vi "New_User Management (Subvi) (TR).vi"() -> ()   [LabVIEW 2009]
uses:
  <vilib>/Utility/file.llb/Read From Spreadsheet File (string).vi
  <vilib>/Utility/file.llb/Write To Spreadsheet File (string).vi
panel:
  in  "Encode/Decode":bool=TRUE
  in  "Magnitude of Shift":u8=22
  in  "Change":bool
  in  "Delete":bool
  in  "Multicolumn Listbox":i32(listbox)
  in  "Yetki":string(combo)="Öğrenci"
  in  "stop":bool
  in  "Create":bool
  in  "Şifre":string
  in  "Kullanıcı Adı":string
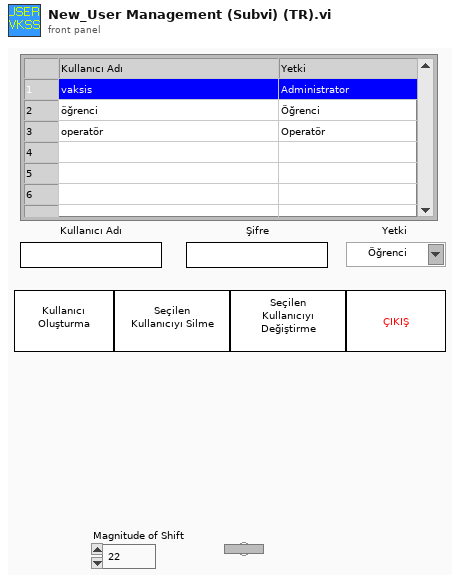
[diagram p1: front panel]
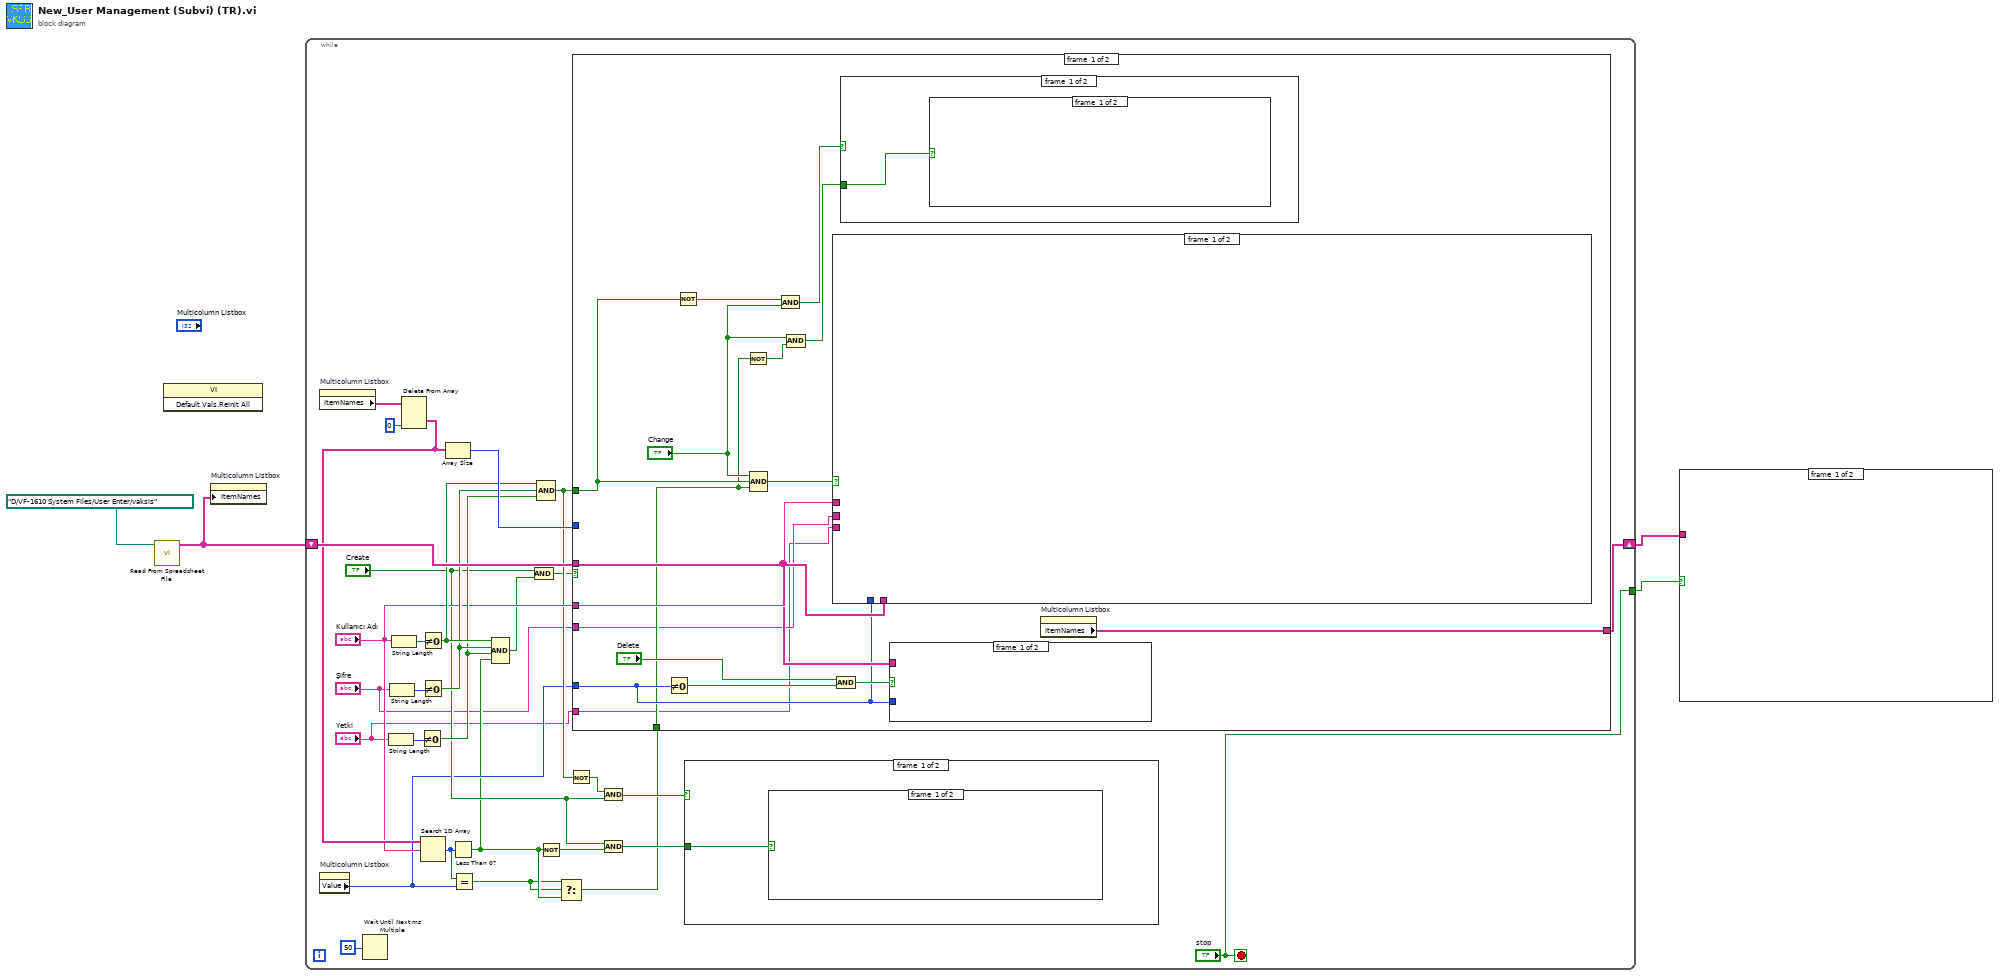
[diagram p0: block diagram]
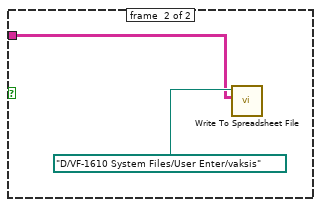
[diagram p2: hidden frame]
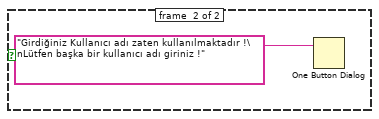
[diagram p3: hidden frame]
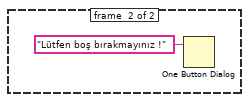
[diagram p4: hidden frame]
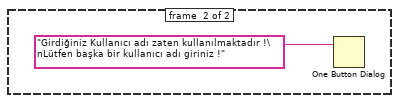
[diagram p5: hidden frame]
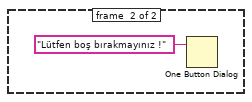
[diagram p6: hidden frame]
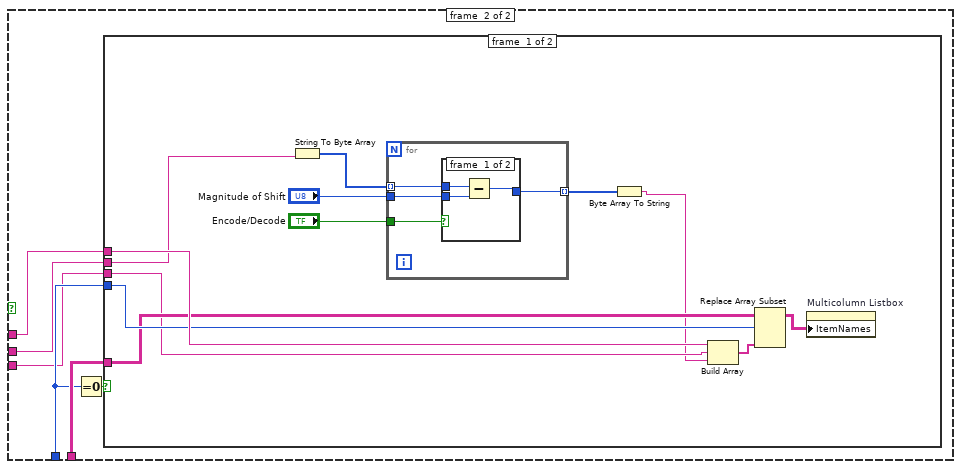
[diagram p7: hidden frame]
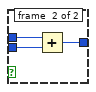
[diagram p8: hidden frame]
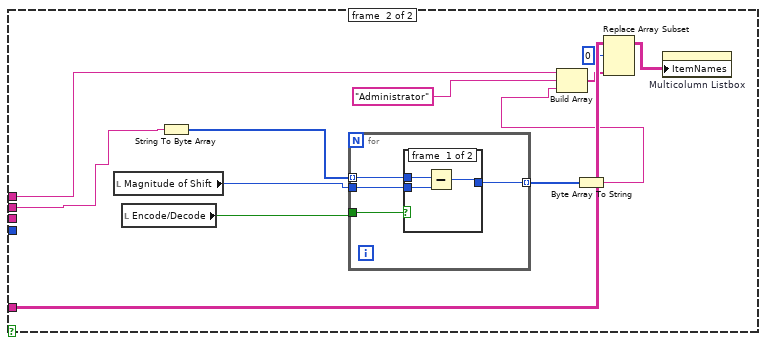
[diagram p9: hidden frame]
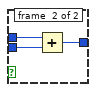
[diagram p10: hidden frame]
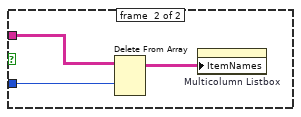
[diagram p11: hidden frame]
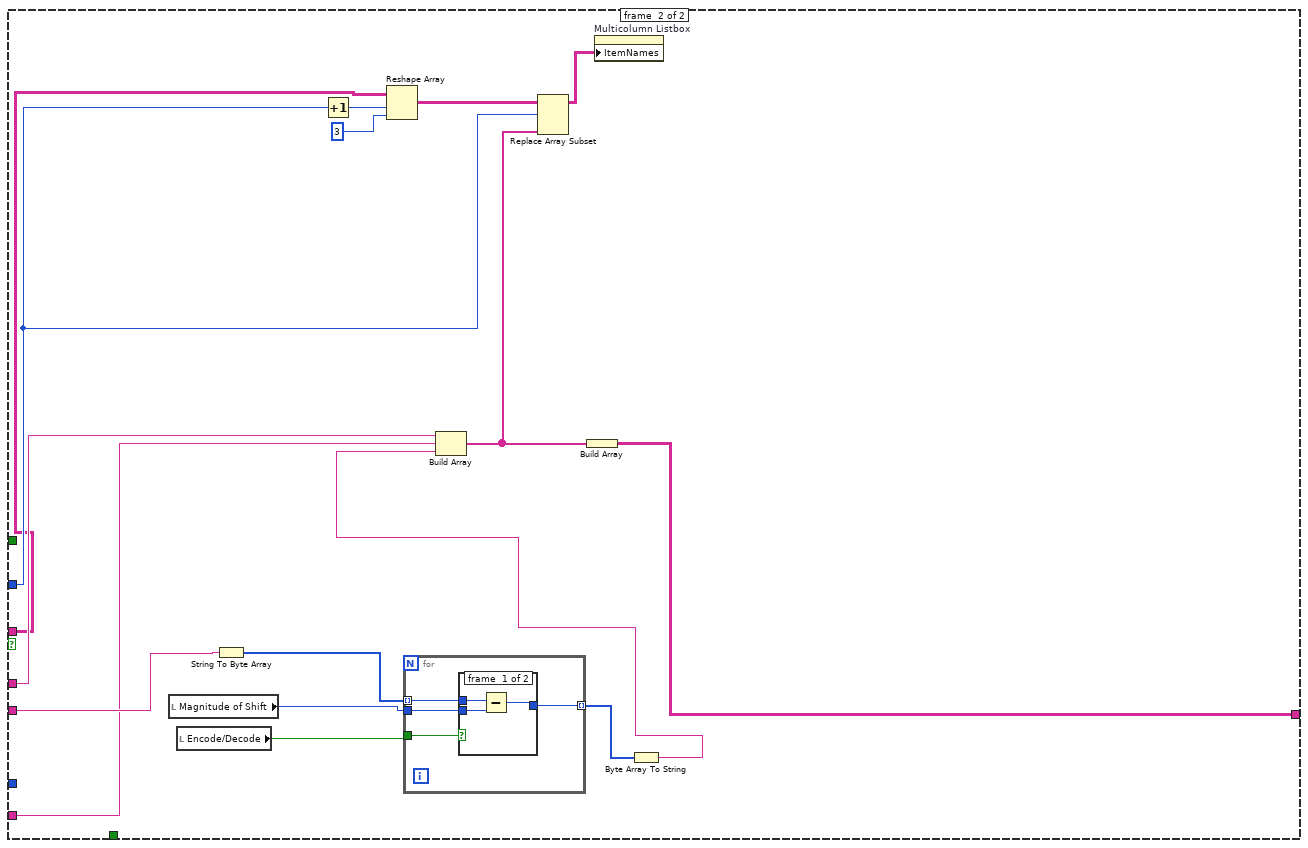
[diagram p12: hidden frame]
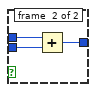
[diagram p13: hidden frame]
diagram:
  n1 = call-poly <vilib>:"Read From Spreadsheet File.vi"("file path (dialog if empty)"=path "D:/VF-1610 System Files/User Enter/vaksis" ("file (use dialog) 2")) -> ("all rows"=w1:string[][])  [unwired: 6 in, 4 out]
  n2 = invoke class="VI" method="Default Vals.Reinit All"() -> ()  [unwired: 3 in, 3 out]
  n3 = property on="Multicolumn Listbox" class="MCListbox (strict)"("ItemNames"=w1) -> ()  [unwired: 2 in, 2 out]
  n4 = while {
    shift-right: [w30] -> w3
    shift-left: w1 -> [w32]
    tunnel: ["stop"] -> w2
    stop <- "stop" stop-if-true
    n5 = property on="Multicolumn Listbox" class="MCListbox (strict)"() -> ("ItemNames"=w25:string[][])  [unwired: 2 in, 2 out]
    n6 = property on="Multicolumn Listbox" class="MCListbox (strict)"() -> ("Value"=w10:i32)  [unwired: 2 in, 2 out]
    n7 = Wait Until Next ms Multiple(millisecond multiple=u32 50) -> ()  [unwired: 1 out]
    n8 = String Length(string="Yetki") -> (length=w28:i32)
    n9 = String Length(string="Şifre") -> (length=w27:i32)
    n10 = String Length(string="Kullanıcı Adı") -> (length=w29:i32)
    n11 = Delete From Array(array=w25, index (col)=0 ("disabled index (col)")) -> (deleted portion=w20:string[])  [unwired: 2 in, 1 out]
    n12 = Not Equal To 0?(x=w28) -> (x != 0?=w21:bool)
    n13 = Not Equal To 0?(x=w29) -> (x != 0?=w23:bool)
    n14 = Not Equal To 0?(x=w27) -> (x != 0?=w22:bool)
    n15 = Search 1D Array(1D array=w20, element="Kullanıcı Adı") -> (index of element=w11:i32)  [unwired: 1 in]
    n16 = Array Size(array=w20) -> (size(s)=w24:i32)
    n17 = Less Than 0?(x=w11) -> (x < 0?=w9:bool)
    n18 = Equal?(x=w11, y=w10) -> (x = y?=w8:bool)
    n19 = Compound Arithmetic op=AND(w23, w22, w21, w9) -> (w13:bool)
    n20 = And(x="Create", y=w13) -> (x .and. y?=w14:bool)
    n21 = Compound Arithmetic op=AND(w23, w22, w21) -> (w18:bool)
    n22 = Not(x=w9) -> (.not. x?=w17:bool)
    n23 = Select(t=w8, s=w8, f=w9) -> (s? t:f=w7:bool)
    n24 = Not(x=w18) -> (.not. x?=w26:bool)
    n25 = case shown="False" w14 {
      tunnel: w24 -> [_ w122]
      tunnel: [w53 w123] -> w30
      tunnel: w32 -> [w52 w119]
      tunnel: "Kullanıcı Adı" -> [w54 w126]
      tunnel: "Yetki" -> [w38 w112]
      tunnel: "Şifre" -> [w39 w113]
      tunnel: w18 -> [w42 _]
      tunnel: w10 -> [w43 _]
      tunnel: w7 -> [w41 _]
      frame #0 {
        n26 = Not Equal To 0?(x=w43) -> (x != 0?=w49:bool)
        n27 = Not(x=w42) -> (.not. x?=w47:bool)
        n28 = Not(x=w41) -> (.not. x?=w40:bool)
        n29 = Compound Arithmetic op=AND("Change", w42, w41) -> (w51:bool)
        n30 = Compound Arithmetic op=AND(w47, "Change") -> (w46:bool)
        n31 = Compound Arithmetic op=AND("Change", w40) -> (w44:bool)
        n32 = case shown="True" w51 {
          tunnel: w52 -> [_ w62]
          tunnel: w54 -> [_ w61]
          tunnel: w39 -> [_ w60]
          tunnel: w43 -> [_ w59]
          tunnel: w38 -> [_ w58]
          frame #0 {
          }
          frame #1 {
            n33 = Equal To 0?(x=w59) -> (x = 0?=w63:bool)
            n34 = case shown="True" w63 {
              tunnel: w61 -> [w73 w93]
              tunnel: w60 -> [w66 w89]
              tunnel: w62 -> [w71 w97]
              tunnel: w59 -> [w72 _]
              tunnel: w58 -> [w65 _]
              frame #0 {
                n35 = String To Byte Array(string=w66) -> (unsigned byte array=w70:u8[])
                n36 = for {
                  tunnel: w70 -> [w79] mode=indexing
                  tunnel: "Magnitude of Shift" -> [w78]
                  tunnel: [w77] -> w68 mode=indexing
                  tunnel: "Encode/Decode" -> [w76]
                  n37 = case shown="False" w76 {
                    tunnel: w79 -> [w81 w85]
                    tunnel: w78 -> [w82 w84]
                    tunnel: [w80 w83] -> w77
                    frame #0 {
                      n38 = Subtract(x=w81, y=w82) -> (x-y=w80:u8)
                    }
                    frame #1 {
                      n39 = Add(x=w85, y=w84) -> (x+y=w83:u8)
                    }
                  }
                }
                n40 = Byte Array To String(unsigned byte array=w68) -> (string=w64:string)
                n41 = Build Array(w73, w65, w64) -> (w75:string[])
                n42 = Replace Array Subset(array=w71, new element=w75, index (row)=w72) -> (w74:string[][])  [unwired: 1 in]
                n43 = property on="Multicolumn Listbox" class="MCListbox (strict)"("ItemNames"=w74) -> ()  [unwired: 2 in, 2 out]
              }
              frame #1 {
                n44 = local read "Magnitude of Shift"() -> (w91:u8)
                n45 = local read "Encode/Decode"() -> (w92:bool)
                n46 = String To Byte Array(string=w89) -> (unsigned byte array=w88:u8[])
                n47 = for {
                  tunnel: w88 -> [w101] mode=indexing
                  tunnel: w91 -> [w100]
                  tunnel: [w99] -> w90 mode=indexing
                  tunnel: w92 -> [w98]
                  n48 = case shown="True" w98 {
                    tunnel: w101 -> [w102 w105]
                    tunnel: w100 -> [w104 w107]
                    tunnel: [w103 w106] -> w99
                    frame #0 {
                      n49 = Subtract(x=w102, y=w104) -> (x-y=w103:u8)
                    }
                    frame #1 {
                      n50 = Add(x=w105, y=w107) -> (x+y=w106:u8)
                    }
                  }
                }
                n51 = Byte Array To String(unsigned byte array=w90) -> (string=w87:string)
                n52 = Build Array(w93, "Administrator" ("element"), w87) -> (w96:string[])
                n53 = Replace Array Subset(array=w97, new element=w96, index (row)=0) -> (w94:string[][])  [unwired: 1 in]
                n54 = property on="Multicolumn Listbox" class="MCListbox (strict)"("ItemNames"=w94) -> ()  [unwired: 2 in, 2 out]
              }
            }
          }
        }
        n55 = Compound Arithmetic op=AND("Delete", w49) -> (w50:bool)
        n56 = case shown="False" w46 {
          tunnel: w44 -> [w55 _]
          frame #0 {
            n57 = case shown="True" w55 {
              frame #0 {
              }
              frame #1 {
                n58 = One Button Dialog(message="Girdiğiniz Kullanıcı adı zaten kullanılmaktadır !\nLütfen başka bir kullanıcı adı giriniz !") -> ()  [unwired: 1 in, 1 out]
              }
            }
          }
          frame #1 {
            n59 = One Button Dialog(message="Lütfen boş bırakmayınız !") -> ()  [unwired: 1 in, 1 out]
          }
        }
        n60 = case shown="True" w50 {
          tunnel: w52 -> [_ w108]
          tunnel: w43 -> [_ w109]
          frame #0 {
          }
          frame #1 {
            n61 = Delete From Array(array=w108, index (row)=w109) -> (array with subset deleted=w110:string[][])  [unwired: 2 in, 1 out]
            n62 = property on="Multicolumn Listbox" class="MCListbox (strict)"("ItemNames"=w110) -> ()  [unwired: 2 in, 2 out]
          }
        }
        n63 = property on="Multicolumn Listbox" class="MCListbox (strict)"() -> ("ItemNames"=w53:string[][])  [unwired: 2 in, 2 out]
      }
      frame #1 {
        n64 = local read "Magnitude of Shift"() -> (w116:u8)
        n65 = local read "Encode/Decode"() -> (w117:bool)
        n66 = String To Byte Array(string=w113) -> (unsigned byte array=w114:u8[])
        n67 = Increment(x=w122) -> (x+1=w125:i32)
        n68 = Reshape Array(w119, w125, 3 ("dimension size")) -> (w118:string[][])
        n69 = for {
          tunnel: w114 -> [w130] mode=indexing
          tunnel: w116 -> [w129]
          tunnel: [w128] -> w115 mode=indexing
          tunnel: w117 -> [w127]
          n70 = case shown="True" w127 {
            tunnel: w130 -> [w131 w134]
            tunnel: w129 -> [w133 w136]
            tunnel: [w132 w135] -> w128
            frame #0 {
              n71 = Subtract(x=w131, y=w133) -> (x-y=w132:u8)
            }
            frame #1 {
              n72 = Add(x=w134, y=w136) -> (x+y=w135:u8)
            }
          }
        }
        n73 = Byte Array To String(unsigned byte array=w115) -> (string=w111:string)
        n74 = Build Array(w126, w112, w111) -> (w124:string[])
        n75 = Replace Array Subset(array=w118, new element=w124, index (row)=w122) -> (w120:string[][])  [unwired: 1 in]
        n76 = Build Array(w124) -> (w123:string[][])
        n77 = property on="Multicolumn Listbox" class="MCListbox (strict)"("ItemNames"=w120) -> ()  [unwired: 2 in, 2 out]
      }
    }
    n78 = And(x=w26, y="Create") -> (x .and. y?=w16:bool)
    n79 = Compound Arithmetic op=AND("Create", w17) -> (w15:bool)
    n80 = case shown="True" w16 {
      tunnel: w15 -> [w35 _]
      frame #0 {
        n81 = case shown="True" w35 {
          frame #0 {
          }
          frame #1 {
            n82 = One Button Dialog(message="Girdiğiniz Kullanıcı adı zaten kullanılmaktadır !\nLütfen başka bir kullanıcı adı giriniz !") -> ()  [unwired: 1 in, 1 out]
          }
        }
      }
      frame #1 {
        n83 = One Button Dialog(message="Lütfen boş bırakmayınız !") -> ()  [unwired: 1 in, 1 out]
      }
    }
  }
  n84 = case shown="True" w2 {
    tunnel: w3 -> [_ w137]
    frame #0 {
    }
    frame #1 {
      n85 = call-poly <vilib>:"Write To Spreadsheet File.vi"("2D data"=w137, "file path (dialog if empty)"=path "D:/VF-1610 System Files/User Enter/vaksis" ("file (use dialog)")) -> ()  [unwired: 6 in, 1 out]
    }
  }
